vi "Lickometer-Init.vi"(7 "Device reference":refnum<vi>, 8 "error in (no error)":errorcluster, 10 "OutputRequest event ref":T1, 11 "InputData reference":refnum<vi>) -> (0 "error out":errorcluster, 2 "OutputRequest (dup)":T1, 3 "InputData (dup)":refnum<vi>)   [LabVIEW 2015]
doc: "Initializes a lickometer device. \nWire its reference to the \"Device reference\" input.\n\nInputData reference: create reference from Main VI\nOutputRequest event ref: get this from Rack-Init\n\nThe outputs are just duplicates to make it easier to call a bunch of Device-Init functions."
uses:
  Typedefs/Lickometer.ctl
  Rack/Typedefs/OutputRequest refnum.ctl
  Rack/Typedefs/OutputRequest.ctl
  Rack/Typedefs/InputData cluster.ctl
  Rack/Methods/Port drivers/DigitalInput-DataCluster.ctl
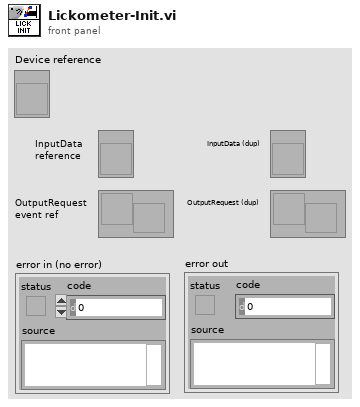
[diagram p1: front panel]
types:
  T1 = typedef "OutputRequest refnum.ctl" = refnum<user-event>
  T2 = typedef "Lickometer.ctl" = cluster{"Settings":cluster{"Min lick duration":u32, "Port name":string, "Port index":i32}, "Lick":bool, "Debouncing":cluster{"Semaphore":T3, "Lick start":u32}, "OutputRequest event ref":T1, "InputData reference":refnum<vi>, "Active hi?":bool}
  T3 = typedef "Semaphore RefNum" = refnum<k1>
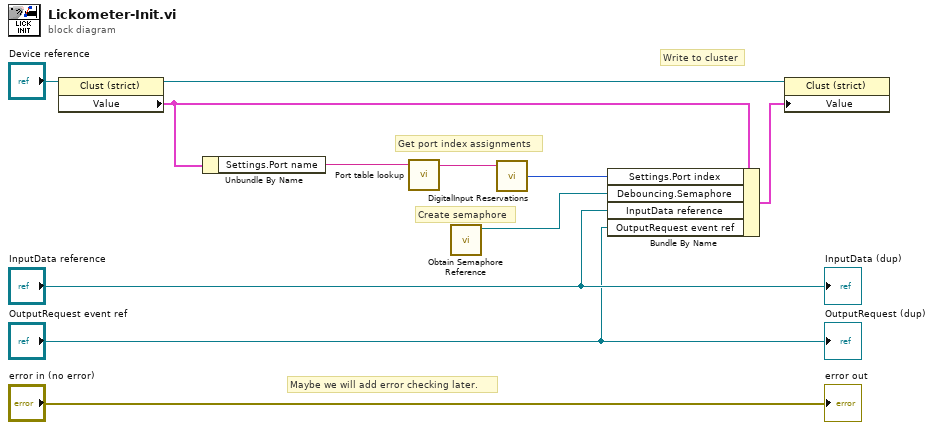
[diagram p0: block diagram]
diagram:
  # "Create semaphore"
  # "Maybe we will add error checking later."
  # "Write to cluster"
  # "Get port index assignments"
  n1 = property class="Clust (strict)"(reference="Device reference") -> (reference out=w10:refnum<vi>, "Value"=w8:T2)  [unwired: 1 in, 1 out]
  n2 = Unbundle By Name(w8) -> ("Settings.Port name"=w7:string)
  n3 = call "Port table lookup.vi"("Port name"=w7) -> ("Line"=w4:tag)  [unwired: 3 in, 1 out]
  n4 = call <vilib>:"Obtain Semaphore Reference.vi"() -> ("semaphore"=w3:T3)  [unwired: 5 in, 2 out]
  n5 = call "DigitalInput Reservations.vi"("Line"=w4) -> ("Index assigned"=w5:i32)  [unwired: 2 in, 2 out]
  n6 = Bundle By Name(cluster=w8, "Settings.Port index"=w5, "Debouncing.Semaphore"=w3, "InputData reference"="InputData reference", "OutputRequest event ref"="OutputRequest event ref") -> (w9:T2)
  n7 = property class="Clust (strict)"(reference=w10, "Value"=w9) -> ()  [unwired: 1 in, 2 out]
  "error out" <- "error in (no error)"
  "OutputRequest (dup)" <- "OutputRequest event ref"
  "InputData (dup)" <- "InputData reference"
